vi "arduino_close_subIV 11-08-2017.vi"(11 "arduino addresses out":T1) -> ()   [LabVIEW 2014]
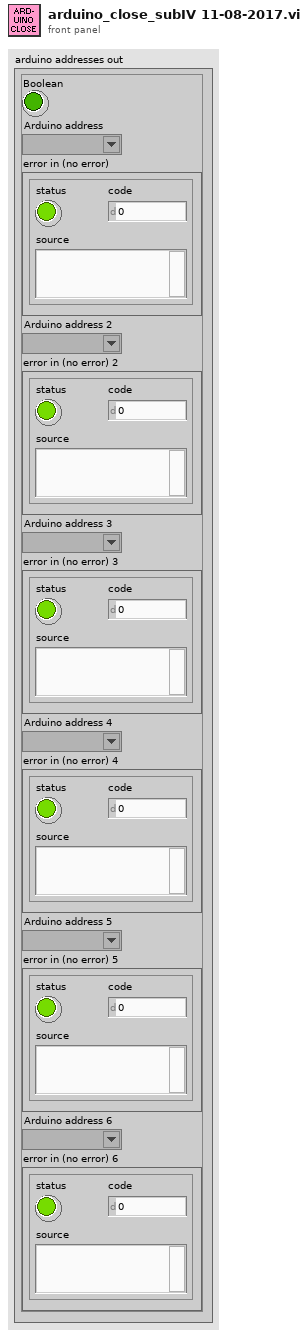
[diagram p1: front panel]
types:
  T1 = cluster{"Boolean":bool, "Arduino address":refnum<visa-resource-name>, "error in (no error)":errorcluster, "Arduino address 2":refnum<visa-resource-name>, "error in (no error) 2":errorcluster, "Arduino address 3":refnum<visa-resource-name>, "error in (no error) 3":errorcluster, "Arduino address 4":refnum<visa-resource-name>, "error in (no error) 4":errorcluster, "Arduino address 5":refnum<visa-resource-name>, "error in (no error) 5":errorcluster, "Arduino address 6":refnum<visa-resource-name>, "error in (no error) 6":errorcluster}
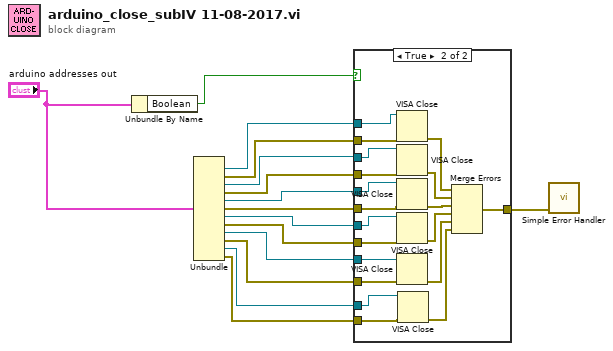
[diagram p0: block diagram]
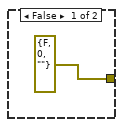
[diagram p2: hidden frame]
diagram:
  n1 = Unbundle By Name("arduino addresses out") -> ("Boolean"=w3:bool)
  n2 = Unbundle("arduino addresses out") -> ("Arduino address"=w15:refnum<visa-resource-name>, "error in (no error)"=w14:errorcluster, "Arduino address 2"=w7:refnum<visa-resource-name>, "error in (no error) 2"=w8:errorcluster, "Arduino address 3"=w9:refnum<visa-resource-name>, "error in (no error) 3"=w10:errorcluster, "Arduino address 4"=w11:refnum<visa-resource-name>, "error in (no error) 4"=w12:errorcluster, "Arduino address 5"=w13:refnum<visa-resource-name>, "error in (no error) 5"=w6:errorcluster, "Arduino address 6"=w5:refnum<visa-resource-name>, "error in (no error) 6"=w1:errorcluster)  [unwired: 1 out]
  n3 = case shown="True" w3 {
    tunnel: w15 -> [_ w28]
    tunnel: w14 -> [_ w27]
    tunnel: w7 -> [_ w26]
    tunnel: w8 -> [_ w25]
    tunnel: w9 -> [_ w24]
    tunnel: w10 -> [_ w23]
    tunnel: w11 -> [_ w22]
    tunnel: w12 -> [_ w21]
    tunnel: w13 -> [_ w20]
    tunnel: w6 -> [_ w19]
    tunnel: w5 -> [_ w18]
    tunnel: [errorcluster {"status"=FALSE, "code"=0, "source"=""} ("error in (no error)") w29] -> w4
    tunnel: w1 -> [_ w17]
    frame False {
    }
    frame True {
      n4 = VISA Close(VISA resource name=w28, error in (no error)=w27) -> (error out=w35:errorcluster)
      n5 = VISA Close(VISA resource name=w26, error in (no error)=w25) -> (error out=w34:errorcluster)
      n6 = VISA Close(VISA resource name=w24, error in (no error)=w23) -> (error out=w33:errorcluster)
      n7 = VISA Close(VISA resource name=w22, error in (no error)=w21) -> (error out=w32:errorcluster)
      n8 = VISA Close(VISA resource name=w20, error in (no error)=w19) -> (error out=w31:errorcluster)
      n9 = VISA Close(VISA resource name=w18, error in (no error)=w17) -> (error out=w30:errorcluster)
      n10 = Merge Errors(w35, w34, w33, w32, w31, w30) -> (w29:errorcluster)
    }
  }
  n11 = call <vilib>:"Simple Error Handler.vi"("error in (no error)"=w4) -> ()  [unwired: 4 in, 5 out]
